vi "DBStringToAssociativeArray.vi"(10 "Raw DB String":string) -> (1 "Values":dbl[](array[numeric]), 2 "Names":string[](array[string]))   [LabVIEW 2012]
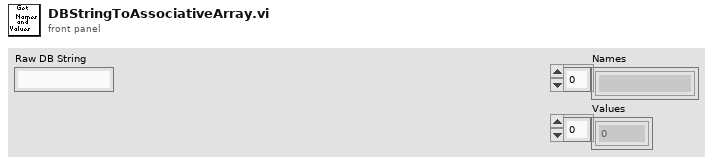
[diagram p1: front panel]
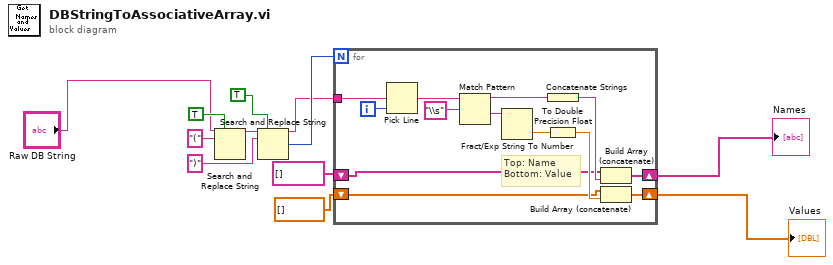
[diagram p0: block diagram]
diagram:
  n1 = Search and Replace String(replace all?=TRUE ("replace all? (F)"), input string="Raw DB String", search string="(") -> (result string=w11:string)  [unwired: 5 in, 3 out]
  n2 = Search and Replace String(replace all?=TRUE ("replace all? (F)"), input string=w11, search string=")") -> (result string=w5:string, number of replacements=w6:i32)  [unwired: 5 in, 2 out]
  n3 = for {
    N: w6 -> [_]
    tunnel: w5 -> [w19]
    shift-right: [w16] -> w2
    shift-left: string[] [] -> [w13]
    shift-right: [w15] -> w1
    shift-left: dbl[] [] -> [w14]
    i -> [w25]
    # "Top: Name\nBottom: Value"
    n4 = Pick Line(multi-line string=w19, line index=w25) -> (output string=w24:string)  [unwired: 1 in]
    n5 = Match Pattern(string=w24, regular expression="\\s") -> (before substring=w21:string, after substring=w22:string)  [unwired: 1 in, 2 out]
    n6 = Fract/Exp String To Number(string=w22) -> (number=w20:dbl)  [unwired: 3 in, 1 out]
    n7 = Concatenate Strings(w21) -> (w18:string)
    n8 = To Double Precision Float(number=w20) -> (double precision float=w17:dbl)
    n9 = Build Array (concatenate)(w13, w18) -> (w16:string[])
    n10 = Build Array (concatenate)(w14, w17) -> (w15:dbl[])
  }
  "Names" <- w2
  "Values" <- w1
